vi "Initialize.vi"(8 "error in (no error)":errorcluster, 10 "Internal?":bool, 11 "Lauda Settings In":T1) -> (0 "error out":errorcluster, 2 "Connection Error":bool, 3 "Lauda Settings Out":T1)   [LabVIEW 2018, in "Lauda TCU.lvlib"]
uses:
  Lauda TCU.lvlib
  Lauda Settings.ctl
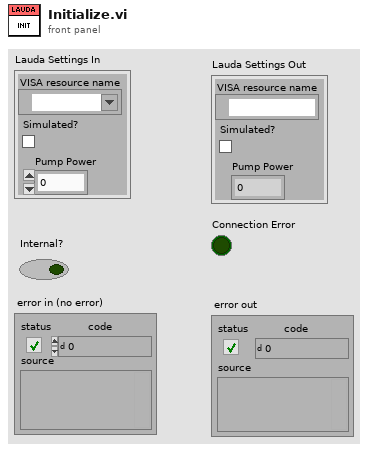
[diagram p1: front panel]
types:
  T1 = typedef "Lauda TCU.lvlib/Lauda Settings.ctl" = cluster{"VISA resource name":refnum<visa-resource-name>, "Simulated?":bool, "Pump Power":i32}
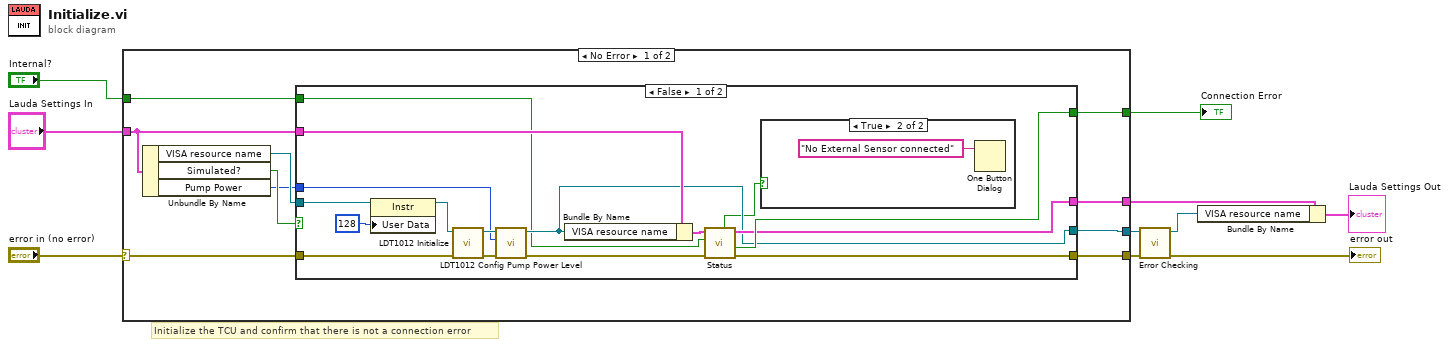
[diagram p0: block diagram]
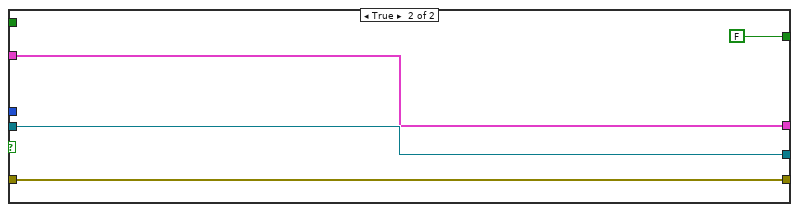
[diagram p3: hidden frame]
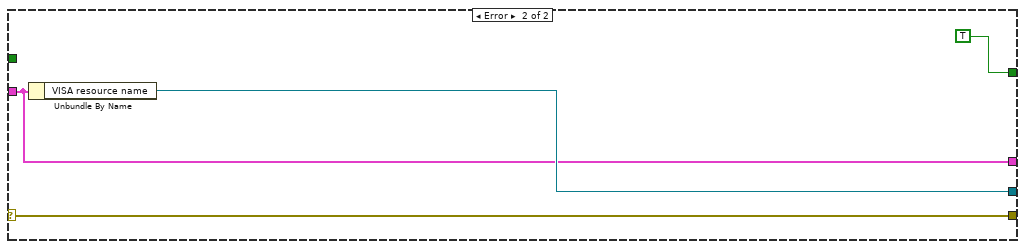
[diagram p4: hidden frame]
diagram:
  # "Initialize the TCU and confirm that there is not a connection error"
  n1 = case shown="No Error" "error in (no error)" {
    selector: "error in (no error)" -> [w20 w45]
    tunnel: "Lauda Settings In" -> [w14 w42]
    tunnel: [w19 w45] -> w8
    tunnel: [w17 w44] -> w9
    tunnel: [w15 TRUE] -> w4
    tunnel: [w13 w42] -> w3
    tunnel: "Internal?" -> [w11 _]
    frame No Error {
      n2 = Unbundle By Name(w14) -> ("VISA resource name"=w18:refnum<visa-resource-name>, "Simulated?"=w16:bool, "Pump Power"=w12:i32)
      n3 = case shown="False" w16 {
        tunnel: w20 -> [w33 w41]
        tunnel: [w34 w41] -> w19
        tunnel: [w27 w40] -> w17
        tunnel: w18 -> [w25 w40]
        tunnel: [w36 FALSE] -> w15
        tunnel: w14 -> [w32 w38]
        tunnel: [w35 w38] -> w13
        tunnel: w12 -> [w29 _]
        tunnel: w11 -> [w21 _]
        frame False {
          n4 = property class="Instr"(reference=w25, "User Data"=u32 128 ("General Settings:User Data")) -> (reference out=w23:refnum<visa-resource-name>)  [unwired: 1 in, 1 out]
          n5 = call "LDT1012 Initialize.vi"("error in (no error)"=w33, "VISA resource name"=w23) -> ("error out"=w28:errorcluster, "VISA session"=w30:refnum<visa-resource-name>)  [unwired: 6 in, 2 out]
          n6 = call "LDT1012 Config Pump Power Level.vi"("error in (no error)"=w28, "Pump Power Level (2: Default)"=w29, "VISA session"=w30) -> ("error out"=w26:errorcluster, "dup VISA session"=w27:refnum<visa-resource-name>)  [unwired: 7 in]
          n7 = Bundle By Name(cluster=w32, "VISA resource name"=w27) -> (w31:T1)
          n8 = call "Status.vi"("error in (no error)"=w26, "Internal?"=w21, "Lauda Settings"=w31) -> ("error out"=w34:errorcluster, "Connection Error"=w36:bool, "Lauda Settings"=w35:T1, "No external Sensor"=w22:bool)  [unwired: 2 in, 3 out]
          n9 = case shown="True" w22 {
            frame False {
            }
            frame True {
              n10 = One Button Dialog(message="No External Sensor connected") -> ()  [unwired: 1 in, 1 out]
            }
          }
        }
        frame True {
        }
      }
    }
    frame Error {
      n11 = Unbundle By Name(w42) -> ("VISA resource name"=w44:refnum<visa-resource-name>)
    }
  }
  "Connection Error" <- w4
  n12 = call "Error Checking.vi"("error in (no error)"=w8, "VISA resource name"=w9) -> ("error out"=→"error out":errorcluster, "VISA resource name"=w6:refnum<visa-resource-name>)  [unwired: 7 in, 1 out]
  n13 = Bundle By Name(cluster=w3, "VISA resource name"=w6) -> (→"Lauda Settings Out":T1)
